vi "String_to_Ch_names.vi"(0 "Spreadsheet string":string) -> (1 "Ch names":string[](array[string]), 2 "Title length (Bytes)":i32, 3 "Title Rows Found?":bool, 4 "String After names":string)   [LabVIEW 2010]
panel:
  out "Data length":i32
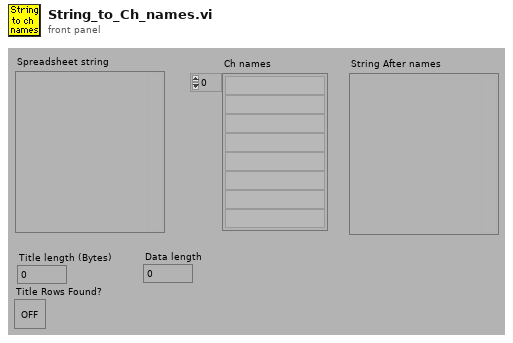
[diagram p1: front panel]
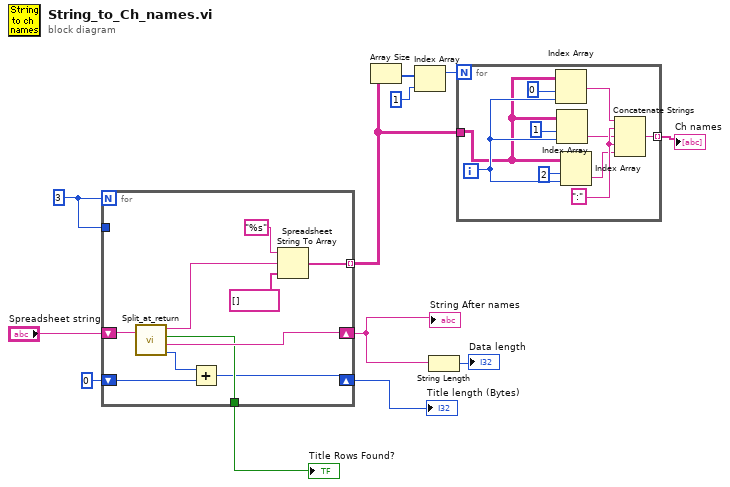
[diagram p0: block diagram]
diagram:
  w12 = 3
  n1 = for {
    N: w12 -> [_]
    shift-right: [w18] -> w9
    shift-left: "Spreadsheet string" -> [w19]
    tunnel: w12 -> [_]
    tunnel: [w17] -> w8
    tunnel: [w16] -> w5 mode=indexing
    shift-right: [w13] -> w1
    shift-left: 0 -> [w14]
    n2 = call "Split_at_return.vi"("String"=w19) -> ("before substring"=w20:string, "Matched?"=w17:bool, "after substring"=w18:string, "offset past match"=w15:i32)  [unwired: 1 in]
    n3 = Add(x=w15, y=w14) -> (x+y=w13:i32)
    n4 = Spreadsheet String To Array(format string="%s", spreadsheet string=w20, array type (2D Dbl)=string[] []) -> (array=w16:string[])  [unwired: 1 out]
  }
  "Title length (Bytes)" <- w1
  "String After names" <- w9
  "Title Rows Found?" <- w8
  n5 = Array Size(array=w5) -> (size(s)=w7:i32[])
  n6 = Index Array(array=w7, index=1 ("Index")) -> (element=w4:i32)
  n7 = String Length(string=w9) -> (length=→"Data length":i32)
  n8 = for {
    N: w4 -> [_]
    tunnel: w5 -> [w27]
    tunnel: [w23] -> w3 mode=indexing
    i -> [w31]
    w32 = ":"
    n9 = Index Array(array=w27, index (row)=0 ("Index"), index (col)=w31) -> (element=w26:string)
    n10 = Index Array(array=w27, index (row)=1 ("Index"), index (col)=w31) -> (element=w25:string)
    n11 = Index Array(array=w27, index (row)=2 ("Index"), index (col)=w31) -> (element=w24:string)
    n12 = Concatenate Strings(w26, w32, w25, w32, w24) -> (w23:string)
  }
  "Ch names" <- w3
